vi "Projekt_Analiza_Obrazkow_Kopia.vi"() -> ()   [LabVIEW 2020]
uses:
  <vilib>/Utility/miscctls.llb/LVPoint32TypeDef.ctl
  Obraz_control.ctl
  <vilib>/vision/NI_Vision_Development_Module.lvlib
panel:
  out "Histogram  Naświetlenia":T1(graph)
  out "Histogram  Naświetlenia":T1(graph)
  out "Szkic":T2(plugin-control)
  out "Szary Odcien":T2(plugin-control)
  in  "Obrazek 4":bool
  out "Obrazek Podstawowy":T3
  out "Prawidłowy zapis \nHEX":string
  out "Liczba do konwersji":u32
  out "B":u8
  out "G":u8
  out "R":u8
  out "Kolor":u32(colorbox)
  out "Kursor - Pozycja":T4
  in  "stop":bool
  out "Pod wzgledem kolorow:":T5
  out "maxIndex B":i32
  out "max B":u32
  out "maxIndex G":i32
  out "max G":u32
  out "maxIndex R":i32
  out "max R":u32
  out "Wartosci Funkcji RGB":T6
  in  "Obrazek 3":bool
  in  "Obrazek 2":bool
  in  "Obrazek 1":bool
  out "Rozdzielczosc":cluster{"Os X":i32, "Os Y":i32}
  in  "Koniec":bool
  out "Histogram RGB":u32[][](graph)
  in  "Szary":bool
  in  "Kolor":bool
  # "Kliknij w przycisk obrazka, aby go wyświetlić.\nProgram umożliwia aktywne pobieranie informacji o kolorze, który znajduje się w obszarze zaznaczenia kursora myszki.\nProgram zczytuje, konwertuje i wyświetla kod HEX, dzięki czemu można dowiedzieć się jaki jest to dokładnie kolor.\nNastępnie wybierz, czy chcesz analizować obrazek pod względem naświetlenia kolorami RGB, czy też  zobaczyć jak \nzmienione zostały kolory w trybie edycji obrazka (wyświetlone zostaną zedytowane kopie)."
  # "Zakonczenie dzialania\nprogramu"
  # "Wniosek: W szkicu zostały użyte tylko kolory czarno-białe.\nNie ma więc tutaj dużego naświetlenia kolorami,\nsą wyróżnione tylko te 2 kolory. Widać to dokładnie na histogramie \nwygenerowanym w obrazku \"szkic\".\nJest to jak najbardziej prawidłowe działanie."
  # "Info:"
  # "Info:"
  # "Pkt"
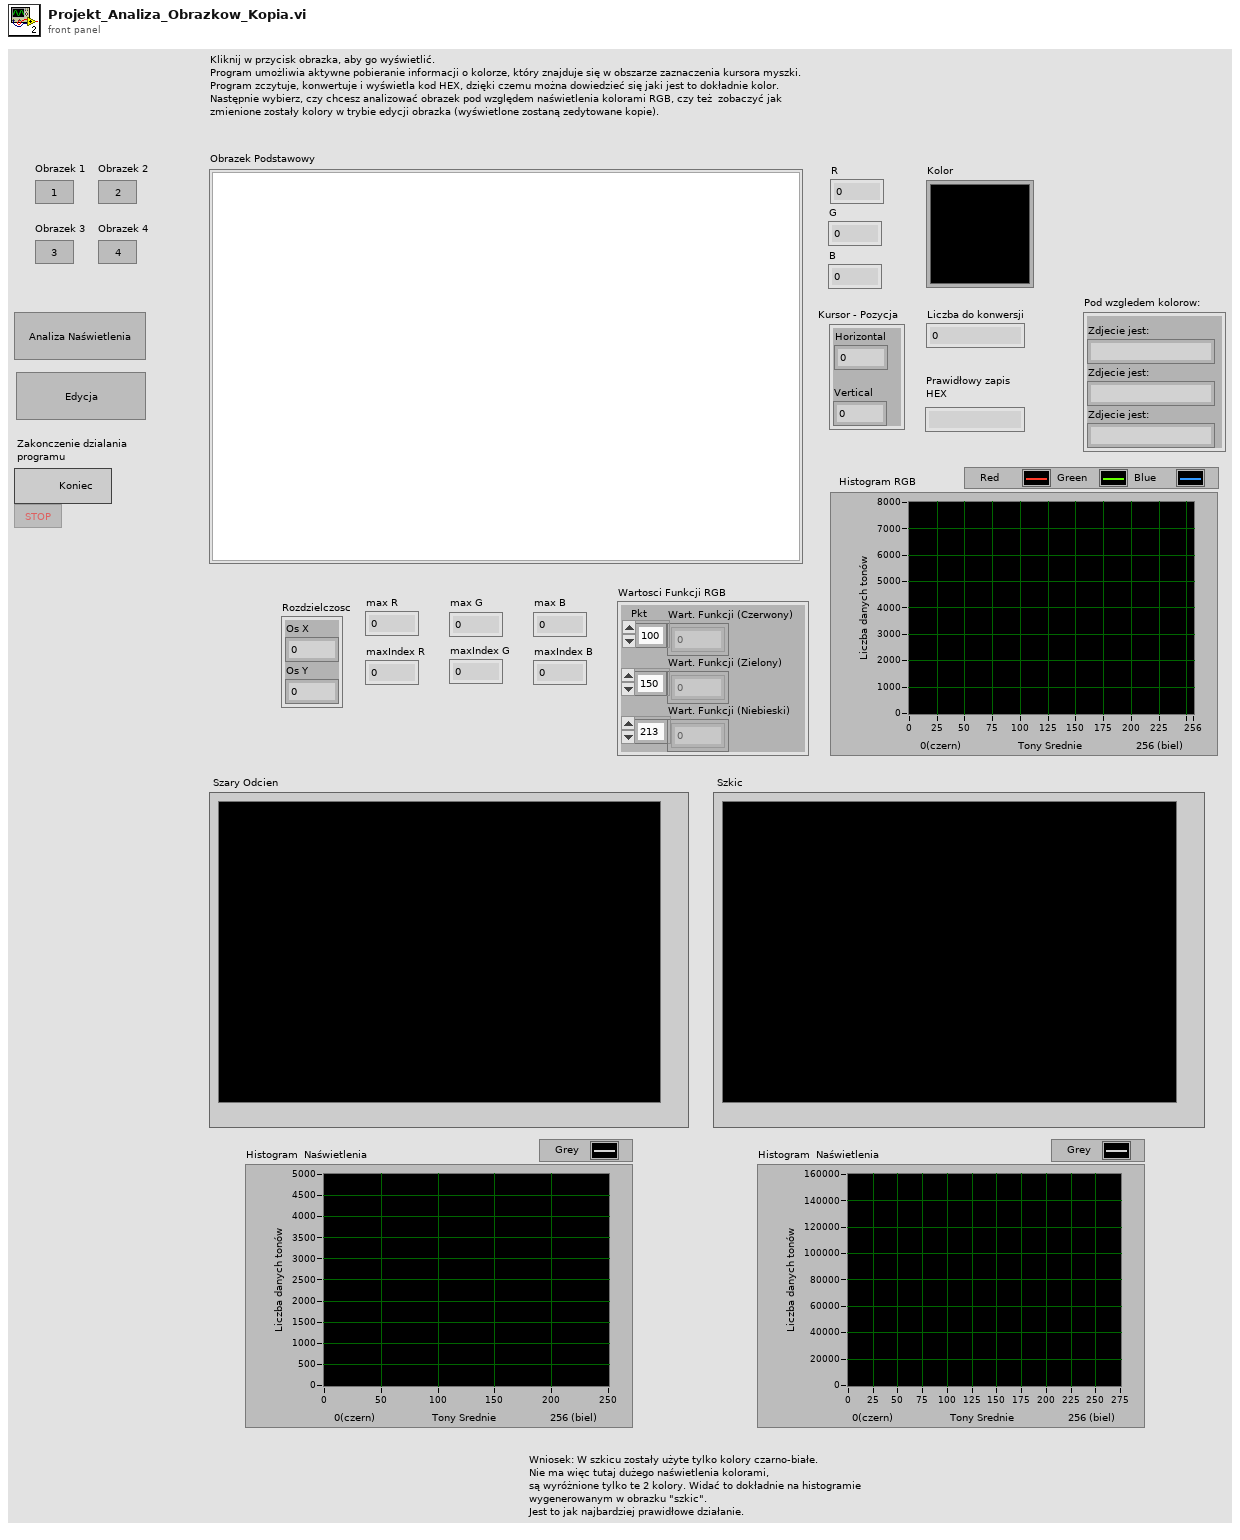
[diagram p1: front panel]
types:
  T1 = cluster{"Starting Value":sgl, "Incremental Value":sgl, "Histogram":u32[]}
  T2 = typedef "IMAQ Image.ctl" = refnum<image>
  T3 = typedef "Obraz_control.ctl" = picture
  T4 = typedef "LVPoint32TypeDef.ctl" = cluster{"Horizontal":i32, "Vertical":i32}
  T5 = cluster{"Zdjecie jest:":string, "Zdjecie jest:":string, "Zdjecie jest:":string}
  T6 = cluster{"Wart. Funkcji (Czerwony) ":u32[], "Wart. Funkcji (Zielony)":u32[], "Wart. Funkcji (Niebieski)":u32[]}
  T7 = typedef "imagedata.ctl" = cluster{"image type":i32, "image depth":i32, "image":u8[], "mask":u8[], "colors":u32[], "Rectangle":cluster{"left":i16, "top":i16, "right":i16, "bottom":i16}}
  T8 = typedef "Image Type" = u32
  T9 = cluster{"Histogram":u32[], "Histogram":u32[], "Histogram":u32[]}
  T10 = cluster{"result string":string, "result string":string, "result string":string}
  T11 = typedef "LVPositionTypeDef.ctl" = cluster{"Left":i32, "Top":i32}
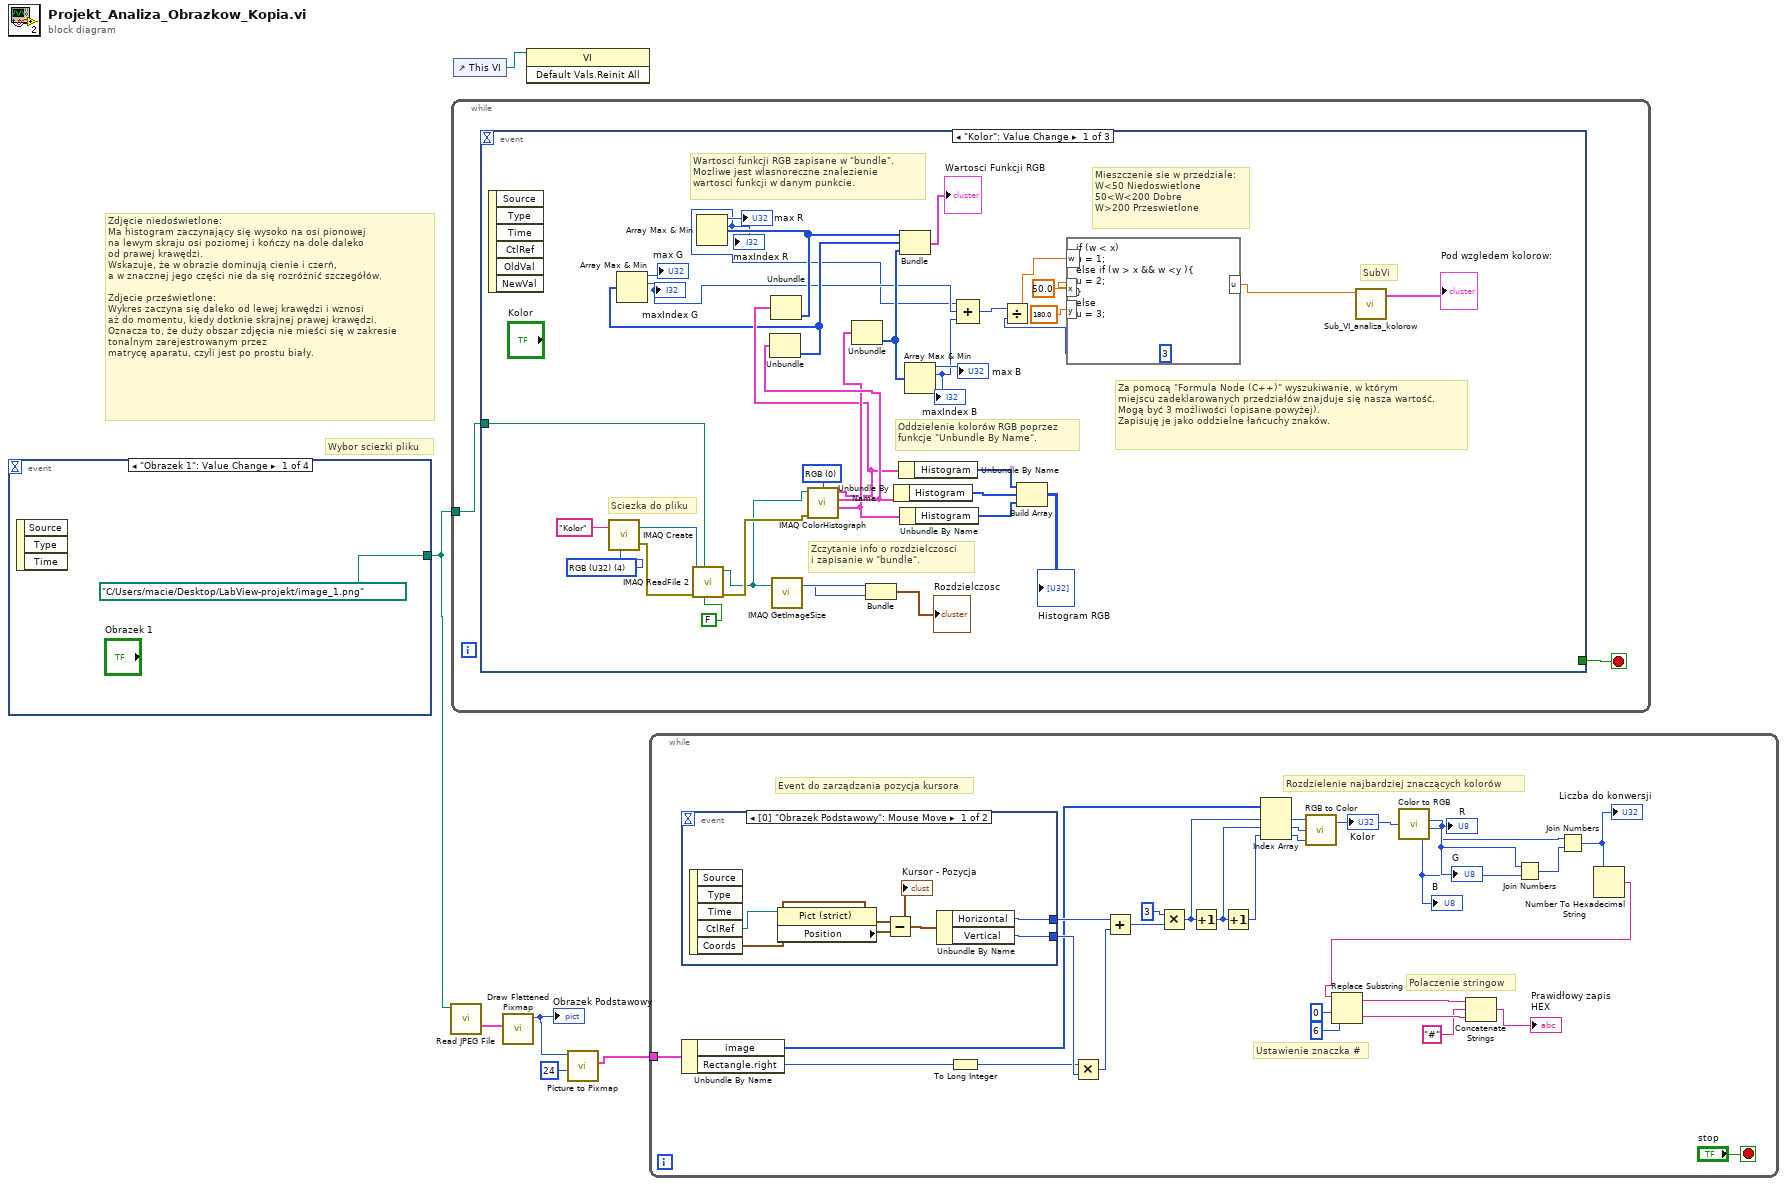
[diagram p0: block diagram]
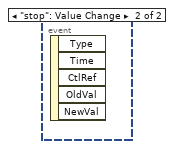
[diagram p2: hidden frame]
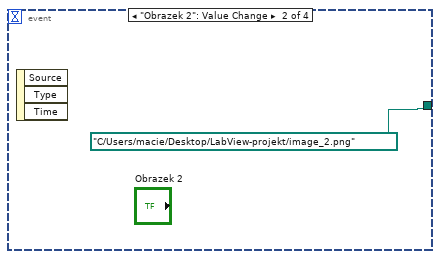
[diagram p3: hidden frame]
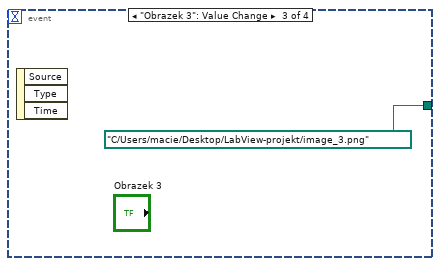
[diagram p4: hidden frame]
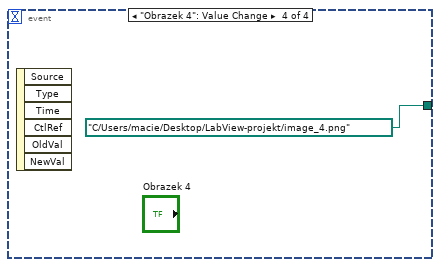
[diagram p5: hidden frame]
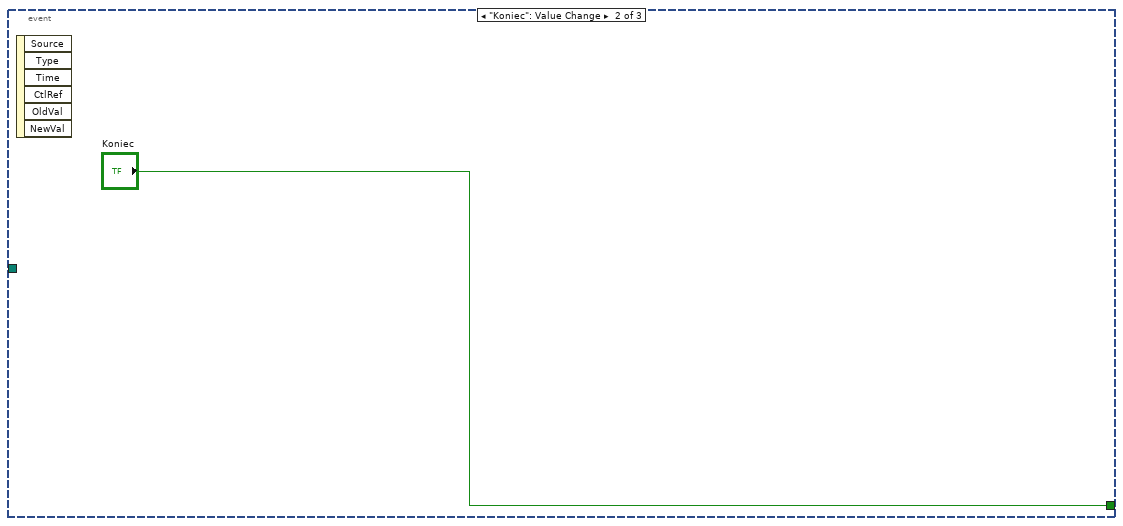
[diagram p6: hidden frame]
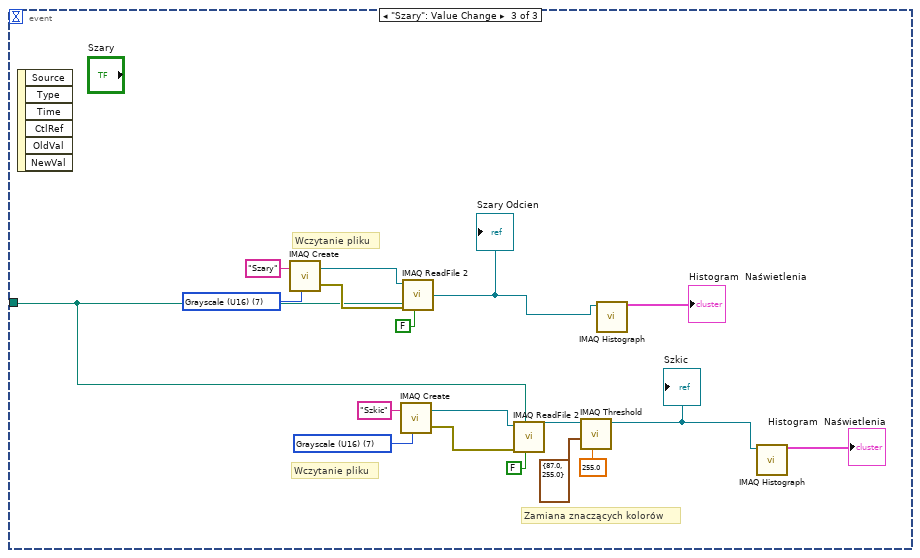
[diagram p7: hidden frame]
diagram:
  # "Zdjęcie niedoświetlone: \nMa histogram zaczynający się wysoko na osi pionowej \nna lewym skraju osi poziomej i kończy na dole daleko \nod prawej krawędzi. \nWskazuje, że w obrazie dominują cienie i czerń, \na w znacznej jego części nie da się rozróżnić szczegółów.\n \nZdjecie prześwietlone: \nWykres zaczyna się daleko od lewej krawędzi i wznosi \naż do momentu, kiedy dotknie skrajnej prawej krawędzi. \nOznacza to, że duży obszar zdjęcia nie mieści się w zakresie tonalnym zarejestrowanym przez \nmatrycę aparatu, czyli jest po prostu biały."
  # "Wybor sciezki pliku"
  n1 = event shown="[0] \"Obrazek 1\": Value Change" {
    selector: _ -> [_ _ _ _]
    dyn-events: _ -> [_ _ _ _]
    timeout: _ -> [_ _ _ _]
    tunnel: [path "C:/Users/macie/Desktop/LabView-projekt/image_1.png" ("File Path") path "C:/Users/macie/Desktop/LabView-projekt/image_2.png" ("File Path") path "C:/Users/macie/Desktop/LabView-projekt/image_3.png" ("File Path") path "C:/Users/macie/Desktop/LabView-projekt/image_4.png" ("File Path")] -> w5
    event "Obrazek 1": Value Change {
      n2 = event-data() -> ()  [unwired: 1 in, 3 out]
    }
    event "Obrazek 2": Value Change {
      n3 = event-data() -> ()  [unwired: 1 in, 3 out]
    }
    event "Obrazek 3": Value Change {
      n4 = event-data() -> ()  [unwired: 1 in, 3 out]
    }
    event "Obrazek 4": Value Change {
      n5 = event-data() -> ()  [unwired: 1 in, 6 out]
    }
  }
  n6 = call <vilib>:"Read JPEG File.vi"("path to JPEG file"=w5) -> ("image data"=w2:T7)  [unwired: 8 in, 2 out]
  n7 = while {
    tunnel: w5 -> [w12]
    stop <- w11 stop-if-true
    n8 = event shown="[0] \"Kolor\": Value Change" {
      selector: _ -> [_ _ _]
      dyn-events: _ -> [_ _ _]
      timeout: _ -> [_ _ _]
      tunnel: [_ "Koniec" _] -> w11
      tunnel: w12 -> [w41 _ w57]
      event "Kolor": Value Change {
        w42 = u16 0 items=["RGB", "HSL", "HSV", "HSI"] ("Color Mode")
        w45 = T8 4 items=["Grayscale (U8)", "Grayscale (I16)", "Grayscale (SGL)", "Complex (CSG)", "RGB (U32)", "HSL (U32)", "RGB (U64)", "Grayscale (U16)"] ("Image Type")
        # "SubVi"
        # "Za pomocą \"Formula Node (C++)\" wyszukiwanie, w którym \nmiejscu zadeklarowanych przedziałów znajduje się nasza wartość.\nMogą być 3 możliwości (opisane powyżej).\nZapisuję je jako oddzielne łańcuchy znaków."
        # "Mieszczenie sie w przedziale: \nW<50 Niedoswietlone\n50<W<200 Dobre\nW>200 Przeswietlone"
        # "Wartosci funkcji RGB zapisane w \"bundle\".\nMozliwe jest wlasnoreczne znalezienie \nwartosci funkcji w danym punkcie."
        # "Zczytanie info o rozdzielczosci \ni zapisanie w \"bundle\"."
        # "Sciezka do pliku"
        # "Oddzielenie kolorów RGB poprzez \nfunkcje \"Unbundle By Name\"."
        n9 = event-data() -> ()  [unwired: 1 in, 6 out]
        n10 = call "IMAQ Create"("Image Name"="Kolor", "Image Type"=w45) -> ("New Image"=w46:T2, "error out"=w47:errorcluster)  [unwired: 3 in]
        n11 = call "IMAQ ReadFile 2"("Use File Path Image Type"=FALSE, "File Path"=w41, "error in (no error)"=w47, "Image"=w46) -> ("error out"=w44:errorcluster, "Image Out"=w32:T2)  [unwired: 3 in, 3 out]
        n12 = call "IMAQ GetImageSize"("Image"=w32) -> ("Y Resolution"=w39:i32, "X Resolution"=w40:i32)  [unwired: 3 in, 1 out]
        n13 = call "IMAQ ColorHistograph"("Color Mode"=w42, "Image Src"=w32, "error in (no error)"=w44) -> ("Red or Hue Histogram Graph"=w35:T1, "Green or Sat Histogram Graph"=w38:T1, "Blue or Luma or Val or Inten Histogram Graph"=w37:T1)  [unwired: 3 in, 1 out]
        n14 = Unbundle(w38) -> ("Histogram"=w28:u32[])  [unwired: 2 out]
        n15 = Array Max & Min(array=w28) -> (max value=→"max G":u32, max index (indices)=w23:i32)  [unwired: 2 out]
        "maxIndex G" <- w23
        n16 = Unbundle(w35) -> ("Histogram"=w30:u32[])  [unwired: 2 out]
        n17 = Array Max & Min(array=w30) -> (max value=→"max R":u32, max index (indices)=w22:i32)  [unwired: 2 out]
        "maxIndex R" <- w22
        n18 = Unbundle(w37) -> ("Histogram"=w25:u32[])  [unwired: 2 out]
        n19 = Bundle("X Resolution"=w40, "Y Resolution"=w39) -> (→"Rozdzielczosc":cluster{"X Resolution":i32, "Y Resolution":i32})  [unwired: 1 in]
        n20 = Unbundle By Name(w38) -> ("Histogram"=w43:u32[])
        n21 = Unbundle By Name(w35) -> ("Histogram"=w34:u32[])
        n22 = Bundle("Histogram"=w30, "Histogram"=w28, "Histogram"=w25) -> (→"Wartosci Funkcji RGB":T9)  [unwired: 1 in]
        n23 = Unbundle By Name(w37) -> ("Histogram"=w33:u32[])
        n24 = Array Max & Min(array=w25) -> (max value=→"max B":u32, max index (indices)=w14:i32)  [unwired: 2 out]
        "maxIndex B" <- w14
        n25 = Compound Arithmetic op=ADD(w22, w23, w14) -> (w21:i32)
        n26 = Divide(x=w21, y=3) -> (x/y=w17:dbl)
        n27 = Build Array(w34, w43, w33) -> (→"Histogram RGB":u32[][])
        n28 = formula code="if (w < x)\nu = 1;\nelse if (w > x && w <y ){\nu = 2;\n}\nelse \nu = 3;"("w"=w17, "x"=50.0 ("input variable"), "y"=180.0 ("input variable")) -> ("u"=w15:dbl)
        n29 = call "Sub_VI_analiza_kolorow.vi"("u"=w15) -> ("Cluster"=→"Pod wzgledem kolorow:":T10)  [unwired: 10 in]
      }
      event "Koniec": Value Change {
        n30 = event-data() -> ()  [unwired: 1 in, 6 out]
      }
      event "Szary": Value Change {
        w61 = T8 7 items=["Grayscale (U8)", "Grayscale (I16)", "Grayscale (SGL)", "Complex (CSG)", "RGB (U32)", "HSL (U32)", "RGB (U64)", "Grayscale (U16)"] ("Image Type")
        w66 = T8 7 items=["Grayscale (U8)", "Grayscale (I16)", "Grayscale (SGL)", "Complex (CSG)", "RGB (U32)", "HSL (U32)", "RGB (U64)", "Grayscale (U16)"] ("Image Type")
        # "Zamiana znaczących kolorów"
        # "Wczytanie pliku"
        # "Wczytanie pliku"
        n31 = event-data() -> ()  [unwired: 1 in, 6 out]
        n32 = call "IMAQ Create"("Image Name"="Szary", "Image Type"=w66) -> ("New Image"=w65:T2, "error out"=w64:errorcluster)  [unwired: 3 in]
        n33 = call "IMAQ Create"("Image Name"="Szkic", "Image Type"=w61) -> ("New Image"=w60:T2, "error out"=w59:errorcluster)  [unwired: 3 in]
        n34 = call "IMAQ ReadFile 2"("Use File Path Image Type"=FALSE, "File Path"=w57, "error in (no error)"=w64, "Image"=w65) -> ("Image Out"=w52:T2)  [unwired: 3 in, 4 out]
        "Szary Odcien" <- w52
        n35 = call "IMAQ ReadFile 2"("Use File Path Image Type"=FALSE, "File Path"=w57, "error in (no error)"=w59, "Image"=w60) -> ("Image Out"=w54:T2)  [unwired: 3 in, 4 out]
        n36 = call "IMAQ Threshold"("Replace Value"=sgl 255.0, "Range"=cluster{"Lower value":sgl, "Upper value":sgl} {"Lower value"=87.0, "Upper value"=255.0}, "Image Src"=w54) -> ("Image Dst Out"=w50:T2)  [unwired: 7 in, 1 out]
        "Szkic" <- w50
        n37 = call "IMAQ Histograph"("Image"=w52) -> ("Histogram Graph"=→"Histogram  Naświetlenia":T1)  [unwired: 7 in, 3 out]
        n38 = call "IMAQ Histograph"("Image"=w50) -> ("Histogram Graph"=→"Histogram  Naświetlenia":T1)  [unwired: 7 in, 3 out]
      }
    }
  }
  n39 = control-ref of="This VI"() -> (w6:refnum<vi>)
  n40 = call <vilib>:"Draw Flattened Pixmap.vi"("image data"=w2) -> ("new picture"=w4:picture)  [unwired: 8 in]
  "Obrazek Podstawowy" <- w4
  n41 = invoke class="VI" method="Default Vals.Reinit All"(reference=w6) -> ()  [unwired: 2 in, 3 out]
  n42 = call <vilib>:"Picture to Pixmap.vi"("depth"=24, "picture"=w4) -> ("image data"=w1:T7)  [unwired: 8 in, 1 out]
  n43 = while {
    tunnel: w1 -> [w93]
    stop <- "stop" stop-if-true
    # "Polaczenie stringow"
    # "Ustawienie znaczka #"
    # "Rozdzielenie najbardziej znaczących kolorów"
    # "Event do zarządzania pozycja kursora"
    n44 = event shown="[0] \"Obrazek Podstawowy\": Mouse Move" {
      selector: _ -> [_ _]
      dyn-events: _ -> [_ _]
      timeout: _ -> [_ _]
      tunnel: [w102 _] -> w96
      tunnel: [w101 _] -> w94
      event Mouse Move {
        n45 = event-data() -> ("CtlRef"=w97:refnum<vi>, "Coords"=w98:T4)  [unwired: 1 in, 3 out]
        n46 = property class="Pict (strict)"(reference=w97) -> ("Position"=w100:T11)  [unwired: 1 in, 2 out]
        n47 = Subtract(x=w98, y=w100) -> (x-y=w99:T4)
        "Kursor - Pozycja" <- w99
        n48 = Unbundle By Name(w99) -> ("Horizontal"=w101:i32, "Vertical"=w102:i32)
      }
      event "stop": Value Change {
        n49 = event-data() -> ()  [unwired: 1 in, 5 out]
      }
    }
    n50 = Unbundle By Name(w93) -> ("image"=w92:u8[], "Rectangle.right"=w84:i16)
    n51 = To Long Integer(number=w84) -> (32bit integer=w83:i32)
    n52 = Multiply(x=w83, y=w96) -> (x*y=w95:i32)
    n53 = Add(x=w94, y=w95) -> (x+y=w91:i32)
    n54 = Multiply(x=3, y=w91) -> (x*y=w85:i32)
    n55 = Increment(x=w85) -> (x+1=w89:i32)
    n56 = Increment(x=w89) -> (x+1=w88:i32)
    n57 = Index Array(array=w92, index #1=w85, index #2=w89, index #3=w88) -> (element #1=w81:u8, element #2=w86:u8, element #3=w82:u8)
    n58 = call <vilib>:"RGB to Color.vi"("B"=w82, "G"=w86, "R"=w81) -> ("Color"=w80:u32)
    "Kolor" <- w80
    n59 = call <vilib>:"Color to RGB.vi"("Color"=w80) -> ("R"=w76:u8, "G"=w79:u8, "B"=w78:u8)  [unwired: 1 out]
    "R" <- w76
    "G" <- w79
    "B" <- w78
    n60 = Join Numbers(hi=w79, lo=w78) -> ((hi.lo)=w77:u16)
    n61 = Join Numbers(hi=w76, lo=w77) -> ((hi.lo)=w75:u32)
    "Liczba do konwersji" <- w75
    n62 = Number To Hexadecimal String(2:w75) -> (0:w71:string)  [unwired: 1 in]
    n63 = Replace Substring(2:6 ("length (len. of substring)"), 3:0 ("offset (0)"), 5:w71) -> (0:w72:string, 1:w73:string)  [unwired: 1 in]
    n64 = Concatenate Strings(w73, "#" ("string"), w72) -> (→"Prawidłowy zapis \nHEX":string)
  }
